vi "Rotation_UnaryMinus.vi"(11 "in ROTATION":T1) -> (3 "out ROTATION":T1)   [LabVIEW 2019, in "PathExecution_Library.lvlib"]
uses:
  ROTATION.ctl
  PathExecution_Library.lvlib
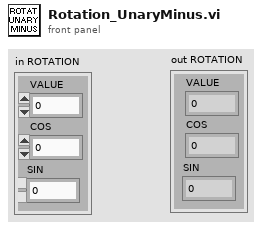
[diagram p1: front panel]
types:
  T1 = typedef "PathExecution_Library.lvlib/ROTATION.ctl" = cluster{"VALUE":dbl, "COS":dbl, "SIN":dbl}
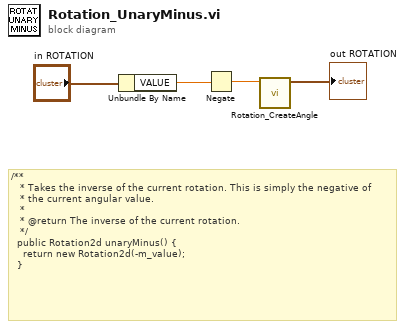
[diagram p0: block diagram]
diagram:
  # "/**\n   * Takes the inverse of the current rotation. This is simply the negative of\n   * the current angular value.\n   *\n   * @return The inverse of the current rotation.\n   */\n  public Rotation2d unaryMinus() {\n    return new Rotation2d(-m_value);\n  }"
  n1 = Unbundle By Name("in ROTATION") -> ("VALUE"=w3:dbl)
  n2 = Negate(x=w3) -> (-x=w2:dbl)
  n3 = call "Rotation_CreateAngle.vi"("Angle"=w2) -> ("ROTATION"=→"out ROTATION":T1)  [unwired: 10 in]
